vi "wordarray to data.vi"(11 "Word array":u16[](array[numeric]) format="%x") -> (3 "Data":u8[](array[numeric]) format="%x")   [LabVIEW 2014]
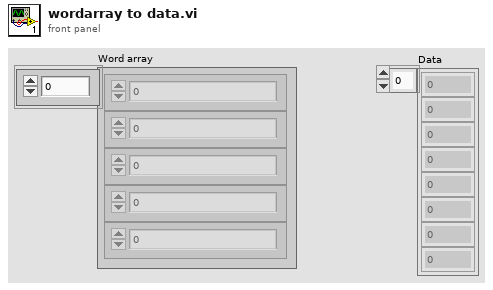
[diagram p1: front panel]
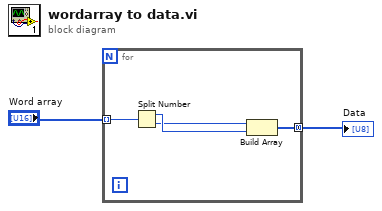
[diagram p0: block diagram]
diagram:
  n1 = for {
    tunnel: "Word array" -> [w6] mode=indexing
    tunnel: [w5] -> w1 mode=concatenating
    n2 = Split Number(x=w6) -> (hi(x)=w4:u8, lo(x)=w3:u8)
    n3 = Build Array(w3, w4) -> (w5:u8[])
  }
  "Data" <- w1
